vi "Configure Display.vi"(8 "error in (no error)":errorcluster, 10 "Display (0: Home Screen)":i32(ring) items=["Home Screen", "Home with Large Readings", "Reading Table", "Graph", "Functions Swipe", "Graph Swipe", "Secondary Swipe", "Setting Swipe", "Statistic Swipe", "User Swipe", "Channel Swipe", "Nonswitch Swipe", "Scan Swipe", "Control Channel", "Settings Channel", "Scan Channel"], 11 "VISA resource name":refnum<visa-resource-name>) -> (0 "error out":errorcluster, 3 "VISA resource name out":refnum<visa-resource-name>)   [LabVIEW 2023, in "Keithley DMM6500 DAQ6500 Series.lvlib"]
doc: "Configures the display settings."
uses:
  <instrlib>/Keithley DMM6500 DAQ6500 Series/Keithley DMM6500 DAQ6500 Series.lvlib
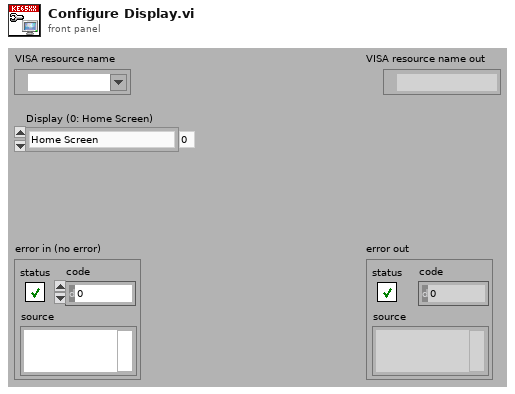
[diagram p1: front panel]
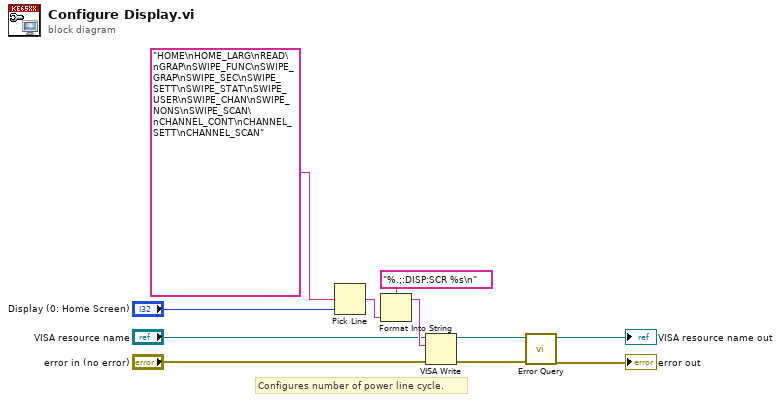
[diagram p0: block diagram]
diagram:
  # "Configures number of power line cycle."
  n1 = Pick Line(multi-line string="HOME\nHOME_LARG\nREAD\nGRAP\nSWIPE_FUNC\nSWIPE_GRAP\nSWIPE_SEC\nSWIPE_SETT\nSWIPE_STAT\nSWIPE_USER\nSWIPE_CHAN\nSWIPE_NONS\nSWIPE_SCAN\nCHANNEL_CONT\nCHANNEL_SETT\nCHANNEL_SCAN", line index="Display (0: Home Screen)") -> (output string=w1:string)  [unwired: 1 in]
  n2 = Format Into String(format string="%.;:DISP:SCR %s\n", w1) -> (resulting string=w10:string)  [unwired: 2 in, 1 out]
  n3 = VISA Write(VISA resource name="VISA resource name", write buffer=w10, error in (no error)="error in (no error)") -> (VISA resource name out=w7:refnum<visa-resource-name>, error out=w6:errorcluster)  [unwired: 1 out]
  n4 = call <instrlib>:"Error Query.vi"("error in (no error)"=w6, "VISA resource name"=w7) -> ("error out"=→"error out":errorcluster, "VISA resource name out"=→"VISA resource name out":refnum<visa-resource-name>)  [unwired: 6 in, 2 out]
